vi "send_data_to_plot.vi"(8 "error in (no error)":errorcluster, 9 "y-value":dbl, 10 "x-value":dbl, 11 "plotname":string) -> (0 "error out":errorcluster)   [LabVIEW 2017]
doc: "sends a data (data x-value,y-value) string to the plot"
uses:
  Classes/Plots/Plots.lvclass
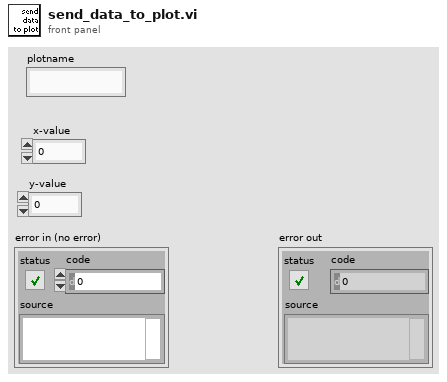
[diagram p1: front panel]
types:
  T1 = cluster{"format string":string, "Variant":variant}
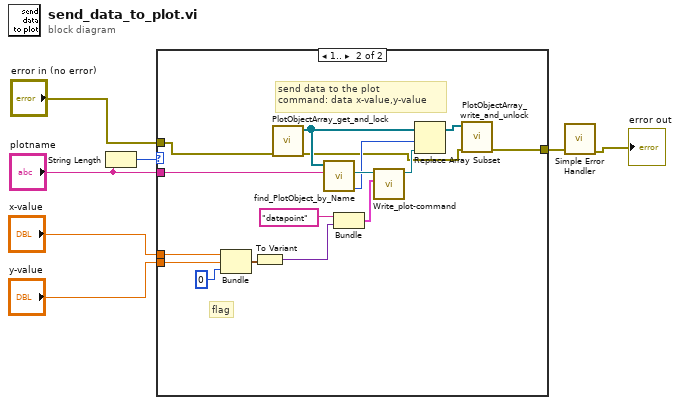
[diagram p0: block diagram]
diagram:
  n1 = String Length(string="plotname") -> (length=w5:i32)
  n2 = case shown="1.." w5 {
    tunnel: "x-value" -> [_ w13]
    tunnel: "y-value" -> [_ w12]
    tunnel: "plotname" -> [_ w19]
    tunnel: "error in (no error)" -> [w8 w18]
    tunnel: [w8 w16] -> w2
    frame 0, Default {
      # "no plotname is given"
    }
    frame 1.. {
      # "flag"
      # "send data to the plot\ncommand: data x-value,y-value"
      n3 = Bundle("x-value"=w13, "y-value"=w12, u8 0) -> (w11:cluster{"x-value":dbl, "y-value":dbl, u8})  [unwired: 1 in]
      n4 = To Variant(anything=w11) -> (Variant=w14:variant)
      n5 = call "PlotObjectArray_get_and_lock.vi"("error in (no error)"=w18) -> ("error out"=w17:errorcluster, "PlotObjects"=w21:refnum<class "Plots.lvclass">[])  [unwired: 9 in]
      n6 = call "find_PlotObject_by_Name.vi"("Plot Name/ID"=w19, "PlotObj Array in"=w21) -> ("index of Object in Array"=w22:i32, "found PlotObj out"=w24:refnum<class "Plots.lvclass">)  [unwired: 6 in, 2 out]
      n7 = Bundle("format string"="datapoint", "Variant"=w14) -> (w10:T1)  [unwired: 1 in]
      n8 = call-dynamic "Write_plot-command.vi"("plot command"=w10, "Plots in"=w24) -> ("Plots out"=w23:refnum<class "Plots.lvclass">)  [unwired: 8 in, 1 out]
      n9 = Replace Array Subset(array=w21, new element=w23, index=w22) -> (w20:refnum<class "Plots.lvclass">[])
      n10 = call "PlotObjectArray_write_and_unlock.vi"("error in (no error)"=w17, "PlotObjects"=w20) -> ("error out"=w16:errorcluster)  [unwired: 9 in]
    }
  }
  n11 = call <vilib>:"Simple Error Handler.vi"("error in (no error)"=w2) -> ("error out"=→"error out":errorcluster)  [unwired: 4 in, 4 out]
